vi "FRC Color Processing RetroTape Example.vi"() -> ()   [LabVIEW 2019]
uses:
  <vilib>/Rock Robotics/WPI/Camera/WPI_CameraSettings Read MJPG.ctl
  <vilib>/Rock Robotics/WPI/Camera/WPI_CameraImageSize.ctl
  Vision Support Code/Camera Types.ctl
  <vilib>/Rock Robotics/WPI/Camera/WPI_CameraExposure Values.ctl
  <vilib>/Rock Robotics/WPI/Camera/WPI_CameraWhite Balance Values.ctl
  <vilib>/vision/NI_Vision_Development_Module.lvlib
panel:
  out "Disqualified":i32=13
  out "Results":T1(array[cluster])=[{"diameter points"={"first point"={"x"=213.0, "y"=163.0}, "projected point"={"x"=293.0, "y"=194.0}}, "Normalized Center"={"x"=0.58125, "y"=0.48750000000000004}, "Overall Score"=61.175669724085026, "Area Score"=96.13589211618256, "Moment Score"=62.73202614698161, "Aspect Score"=24.659090909090907, "Distance (ft)"=4.347709612348454, "Upper Goal"=FALSE}, {"diameter points"={"first point"={"x"=243.0, "y"=142.0}, "projected point"={"x"=266.0, "y"=171.0}}, "Normalized Center"={"x"=0.5906250000000002, "y"=0.3041666666666667}, "Overall Score"=74.56623386292142, "Area Score"=82.18546637744035, "Moment Score"=61.2760810611263, "Aspect Score"=80.23715415019763, "Distance (ft)"=15.122468216864188, "Upper Goal"=FALSE}] {"Normalized Center"."x" format="%#_2g"; "Normalized Center"."y" format="%#_2g"; "Overall Score" format="%#_2g"; "Distance (ft)" format="%#_3g"; "Area Score" format="%#_2g"; "Moment Score" format="%#_2g"; "Aspect Score" format="%#_2g"}
  in  "Size Limit %":dbl=0.04 min=0.0 max=100.0 step=0.01 format="%#_13g"
  out "Instructions:":string="Instructions:\nUse Source to load image files from a directory, or use a USB or IP camera connected to your laptop. Use Camera Settings 1 and 2 to achieve a dark image with bright and colorful stripes.\nLED Color can encoded as HSL or related color modes. Calibrate to the same color as the strips being reflected to the camera.\nClick and draw a line in Original Image to auto-calibrate the LED Color. You may want to widen and tweak Sat and Val by hand.\nThe Annotate button affects drawing a rectangle around the stripes and labeling it with a distance in ft. Distance relies on knowing the Camera Type and lens calibration (it looks up the lens view angle).\n\nAdjust Score Cutoff to make the code more or less picky. If the color is not very unique, you may need to increase the number of particles considered. The diagram uses a Size Limit to ignore colored things that are too small. You may need to adjust it if you are targetting from far away.\n\nResults give you the distance to the target, the center and box in a normalized (-1 to 1) and pixel coordinates.\n\nBe sure to read about setting camera exposure and brightness to help simplify your image and acquire color saturated images.\n\nThere are lots of comments on the diagram to explain the code."
  in  "Color Mode":u16(ring)=2 items=["RGB", "HSL", "HSV", "HSI"]
  in  "Particle Count":i32=5
  in  "Score Threshold %":dbl=75.0
  in  "Std Devs for Calibration":cluster{"H":dbl, "S":dbl, "V":dbl}={"H"=4.0, "S"=8.0, "V"=8.0}
  in  "Camera Type (for distance)":T2=enum."MS HD3000 square"
  in  "image files":string[](array[string])=["BlueGoal-060in-Center.jpg", "BlueGoal-084in-Center.jpg", "BlueGoal-108in-Center.jpg", "BlueGoal-132in-Center.jpg", "BlueGoal-156in-Center.jpg", "BlueGoal-156in-Left.jpg", "BlueGoal-180in-Center.jpg", "BlueGoal-224in-Center.jpg", "BlueGoal-228in-ProtectedZone.jpg", "BlueGoal-330in-ProtectedZone.jpg", "BlueGoal-Far-ProtectedZone.jpg", "RedLoading-016in-Down.jpg", "RedLoading-030in-Down.jpg", "RedLoading-048in-Down.jpg", "RedLoading-048in.jpg", "RedLoading-060in.jpg", "RedLoading-084in.jpg", "RedLoading-108in.jpg"]
  in  "Source":enum32{"Files", "Camera"}(tab)=enum."Camera"
  in  "Images":i32(listbox)
  in  "Folder Location":path=path "C:/Users/5052r/Downloads/2020 Vision Example/Dark Images"
  in  "Camera Settings 1":T3={"fps"=20, "compression"=30, "Image Size"=enum."320x240", "Config Shown"=FALSE}
  in  "Camera Address":string="USB 0"
  in  "Camera Settings 2":T7={"Exposure"=enum."Auto", "Exposure (%)"=50.0, "Brightness"=50, "White Balance"=enum."Auto", "Color Temp (K)"=0.0} {"Brightness" min=0 max=100}
  in  "Annotate":bool=TRUE
  out "Qualified":i32=5
  in  "LED Color Range":T8={"Hue"={14.360681298918061, 47.91090746924753}, "Sat"={75.89285714285714, 255.0}, "Val"={97.14285714285714, 251.32874298095703}} {"Hue" scale=0.0..255.0 scale format="%#_3g"}
  out "Mask":T9(plugin-control)
  out "Original Image":T9(plugin-control)
  # "Limits"
  # "Particle Results"
  # "Good target"
  # "Disqualified"
  # "Distance (ft)"
  # "Scores"
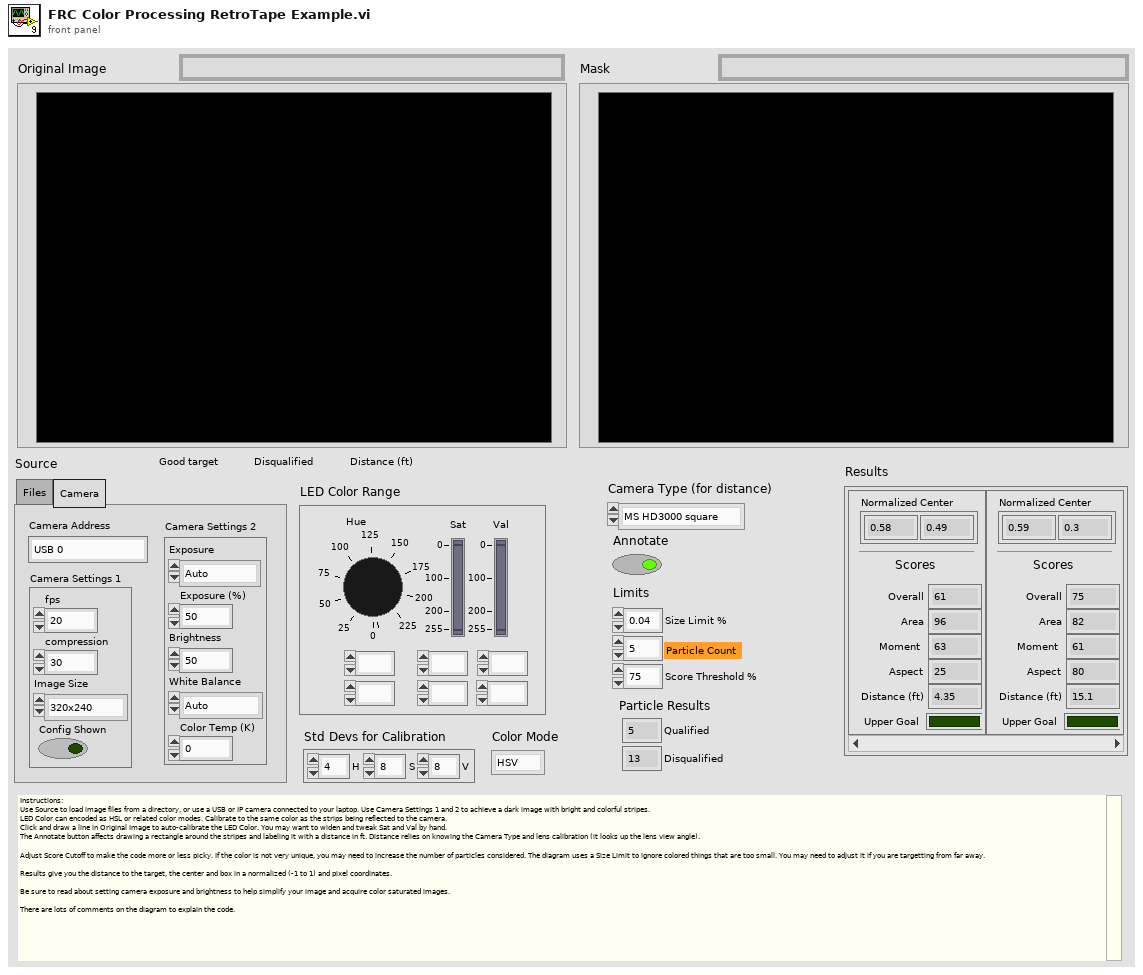
[diagram p1: front panel]
types:
  T1 = cluster{"diameter points":cluster{"first point":cluster{"x":dbl, "y":dbl}, "projected point":cluster{"x":dbl, "y":dbl}}, "Normalized Center":cluster{"x":dbl, "y":dbl}, "Overall Score":dbl, "Area Score":dbl, "Moment Score":dbl, "Aspect Score":dbl, "Distance (ft)":dbl, "Upper Goal":bool}[]
  T2 = typedef "Camera Types.ctl" = enum16{"206", "1011", "1013", "MS HD3000 square", "MS HD3000 640x480"}
  T3 = typedef "WPI_CameraSettings Read MJPG.ctl" = cluster{"fps":i32, "compression":i32, "Image Size":T4, "Config Shown":bool}
  T4 = typedef "WPI_CameraImageSize.ctl" = enum16{"640x480", "320x240", "160x120", "Custom"}
  T5 = typedef "WPI_CameraExposure Values.ctl" = enum16{"Auto", "Flicker-free 50 Hz", "Flicker-free 60 Hz", "Hold current", "Custom"}
  T6 = typedef "WPI_CameraWhite Balance Values.ctl" = enum16{"Auto", "Fixed indoor", "Fixed outdoor 1", "Fixed outdoor 2", "Fixed fluorescent 1", "Fixed fluorescent 2", "Hold current", "Custom"}
  T7 = cluster{"Exposure":T5, "Exposure (%)":dbl, "Brightness":i32, "White Balance":T6, "Color Temp (K)":dbl}
  T8 = cluster{"Hue":cluster{dbl, dbl}, "Sat":cluster{dbl, dbl}, "Val":cluster{dbl, dbl}}
  T9 = typedef "IMAQ Image.ctl" = refnum<image>
  T10 = typedef "Particle Parameters" = i32
  T11 = typedef "Image Type" = u32
  T12 = enum32{"AutoM", "Close", "Dilate", "Erode", "Gradient", "Gradient out", "Gradient in", "Hit miss", "Open", "PClose", "POpen", "Thick", "Thin"}
  T13 = cluster{cluster{dbl, dbl}, cluster{dbl, dbl}, cluster{dbl, dbl}}
  T14 = cluster{"remainder":i32, "size":bool, "count":bool}
  T15 = typedef "Target Fields.ctl" = cluster{"diameter points":cluster{"first point":cluster{"x":dbl, "y":dbl}, "projected point":cluster{"x":dbl, "y":dbl}}, "normalized center":cluster{"x":dbl, "y":dbl}, "Overall Score":dbl, "Area Score":dbl, "Moment Score":dbl, "Aspect Score":dbl, "Distance (ft)":dbl, "Upper Goal":bool}
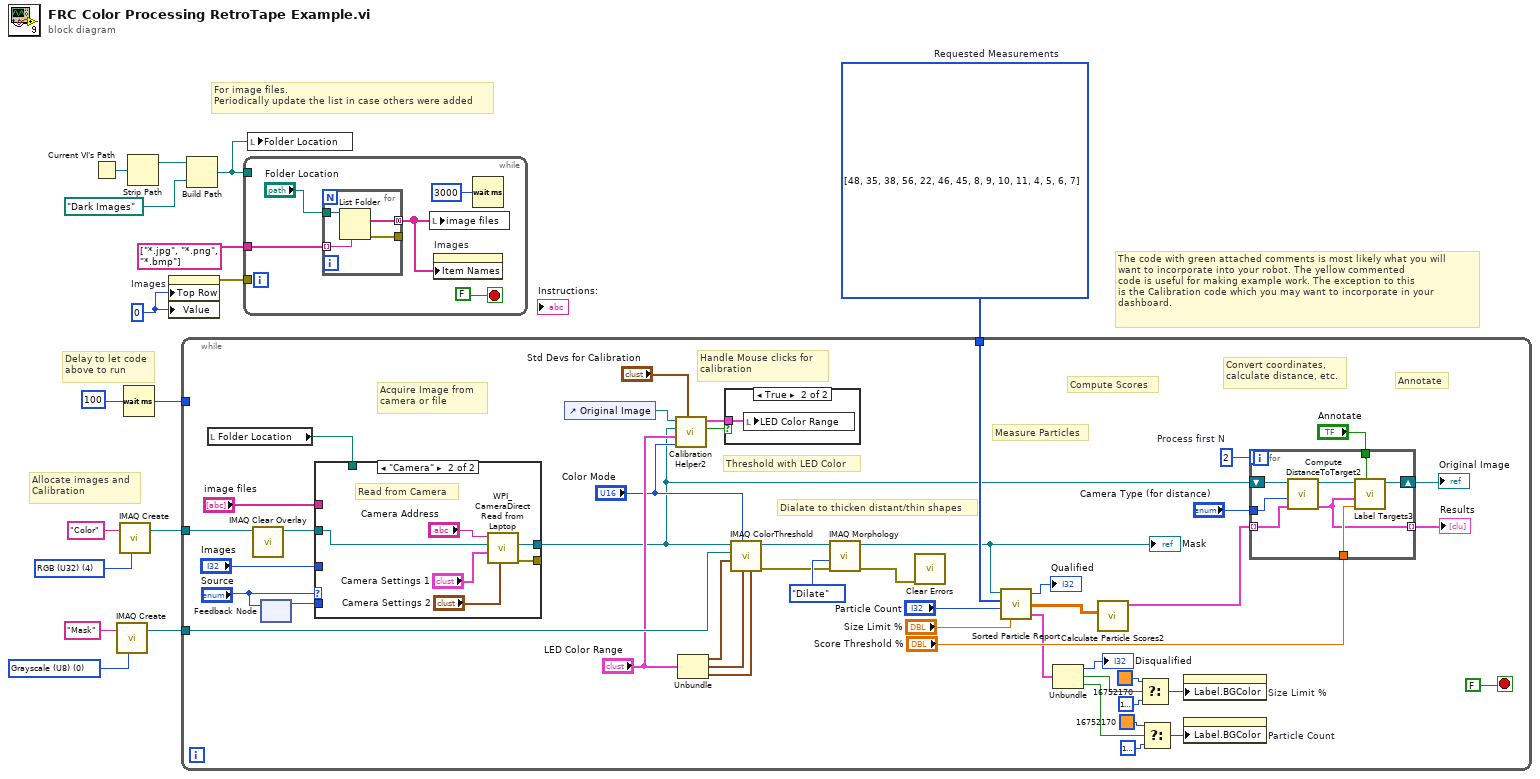
[diagram p0: block diagram]
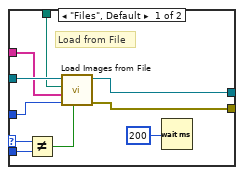
[diagram p3: hidden frame]
diagram:
  w6 = u32 0 ("milliseconds to wait")
  w11 = T10[] [48, 35, 38, 56, 22, 46, 45, 8, 9, 10, 11, 4, 5, 6, 7] items=["Center of Mass X", "Center of Mass Y", "First Pixel X", "First Pixel Y", "Bounding Rect Left", "Bounding Rect Top", "Bounding Rect Right", "Bounding Rect Bottom", "Max Feret Diameter Start X", "Max Feret Diameter Start Y", "Max Feret Diameter End X", "Max Feret Diameter End Y", "Max Horiz. Segment Length Left", "Max Horiz. Segment Length Right", "Max Horiz. Segment Length Row", "-", "Bounding Rect Width", "Bounding Rect Height", "Bounding Rect Diagonal", "Perimeter", "Convex Hull Perimeter", "Holes' Perimeter", "Max Feret Diameter", "Equivalent Ellipse Major Axis", "Equivalent Ellipse Minor Axis", "Equivalent Ellipse Minor Axis (Feret)", "Equivalent Rect Long Side", "Equivalent Rect Short Side", "Equivalent Rect Diagonal", "Equivalent Rect Short Side (Feret)", "Average Horiz. Segment Length", "Average Vert. Segment Length", "Hydraulic Radius", "Waddel Disk Diameter", "-", "Area", "Holes' Area", "Particle & Holes' Area", "Convex Hull Area", "Image Area", "-", "Number of Holes", "Number of Horiz. Segments", "Number of Vert. Segments", "-", "Orientation", "Max Feret Diameter Orientation", "-", "% Area/Image Area", "% Area/(Particle & Holes' Area)", "Ratio of Equivalent Ellipse Axes", "Ratio of Equivalent Rect Sides", "-", "Elongation Factor", "Compactness Factor", "Heywood Circularity Factor", "Type Factor", "-", "Sum X", "Sum Y", "Sum XX", "Sum XY", "Sum YY", "Sum XXX", "Sum XXY", "Sum XYY", "Sum YYY", "-", "Moment of Inertia XX", "Moment of Inertia XY", "Moment of Inertia YY", "Moment of Inertia XXX", "Moment of Inertia XXY", "Moment of Inertia XYY", "Moment of Inertia YYY", "Norm. Moment of Inertia XX", "Norm. Moment of Inertia XY", "Norm. Moment of Inertia YY", "Norm. Moment of Inertia XXX", "Norm. Moment of Inertia XXY", "Norm. Moment of Inertia XYY", "Norm. Moment of Inertia YYY", "Hu Moment 1", "Hu Moment 2", "Hu Moment 3", "Hu Moment 4", "Hu Moment 5", "Hu Moment 6", "Hu Moment 7"]  # Requested Measurements
  w14 = T11 0 items=["Grayscale (U8)", "Grayscale (I16)", "Grayscale (SGL)", "Complex (CSG)", "RGB (U32)", "HSL (U32)", "RGB (U64)", "Grayscale (U16)"] ("Image Type")
  w15 = T11 4 items=["Grayscale (U8)", "Grayscale (I16)", "Grayscale (SGL)", "Complex (CSG)", "RGB (U32)", "HSL (U32)", "RGB (U64)", "Grayscale (U16)"] ("Image Type")
  # "Delay to let code\nabove to run"
  # "The code with green attached comments is most likely what you will\nwant to incorporate into your robot. The yellow commented\ncode is useful for making example work. The exception to this\nis the Calibration code which you may want to incorporate in your\ndashboard."
  # "For image files.\nPeriodically update the list in case others were added"
  # "Allocate images and\nCalibration"
  n1 = Current VI's Path() -> (path=w10:path)
  n2 = call "IMAQ Create"("Image Name"="Mask", "Image Type"=w14) -> ("New Image"=w12:T9)  [unwired: 2 in, 2 out]
  n3 = call "IMAQ Create"("Image Name"="Color", "Image Type"=w15) -> ("New Image"=w4:T9)  [unwired: 2 in, 2 out]
  n4 = Wait (ms)(milliseconds to wait=u32 100) -> (millisecond timer value=w2:u32)
  n5 = Strip Path(path=w10) -> (stripped path=w8:path)  [unwired: 1 out]
  n6 = property on="Images" class="LstBox (strict)"("Top Row"=w6, "Value"=w6) -> (error out=w7:errorcluster)  [unwired: 2 in, 1 out]
  n7 = while {
    tunnel: w4 -> [w37]
    tunnel: w12 -> [w60]
    tunnel: w11 -> [w56]
    tunnel: w2 -> [_]
    stop <- FALSE stop-if-true
    w39 = 2  # Process first N
    # "Dialate to thicken distant/thin shapes"
    # "Handle Mouse clicks for\ncalibration"
    # "Measure Particles"
    # "Convert coordinates,\ncalculate distance, etc."
    # "Annotate"
    # "Compute Scores"
    # "Threshold with LED Color"
    # "Acquire Image from\ncamera or file"
    n8 = local read "Folder Location"() -> (w47:path)
    n9 = call "IMAQ Clear Overlay"("Image"=w37) -> ("Image Out"=w36:T9)  [unwired: 2 in, 8 out]
    n10 = feedback #1() -> (w45:enum32{"Files", "Camera"})  [unwired: 1 in]
    n11 = feedback-in #1("Source") -> ()
    n12 = case shown="\"Camera\"" "Source" {
      selector: "Source" -> [w74 _]
      tunnel: [w80 w87] -> _
      tunnel: [w81 w86] -> w38
      tunnel: w36 -> [w79 w85]
      tunnel: "image files" -> [w76 _]
      tunnel: "Images" -> [w78 _]
      tunnel: w47 -> [w77 _]
      tunnel: w45 -> [w73 _]
      frame "Files", Default {
        # "Load from File"
        n13 = Not Equal?(x=w74, y=w73) -> (x != y?=w72:bool)
        n14 = call "Load Images from File.vi"("Force Load"=w72, "Images"=w78, "image files"=w76, "Folder Location"=w77, "Refnum in"=w79) -> ("error out"=w80:errorcluster, "Refnum out"=w81:T9)  [unwired: 4 in, 1 out]
        n15 = Wait (ms)(milliseconds to wait=u32 200 ("delay (ms)")) -> ()  [unwired: 1 out]
      }
      frame "Camera" {
        # "Read from Camera"
        n16 = call <vilib>:"WPI_CameraDirect Read from Laptop.vi"("Camera Settings 2"="Camera Settings 2", "Camera Settings"="Camera Settings 1", "Image"=w85, "address"="Camera Address") -> ("error out"=w87:errorcluster, "Image Out"=w86:T9)  [unwired: 6 in]
      }
    }
    n17 = control-ref of="Original Image"() -> (w52:refnum<vi>)
    n18 = call "Calibration Helper2.vi"("Std Devs"="Std Devs for Calibration", "Color Mode"="Color Mode", "Color Components"="LED Color Range", "Image"=w38, "Image Ctl Refnum"=w52) -> ("Changed"=w51:bool, "output color"=w50:T13)  [unwired: 5 in]
    n19 = Unbundle("LED Color Range") -> ("Hue"=w59:cluster{dbl, dbl}, "Sat"=w58:cluster{dbl, dbl}, "Val"=w57:cluster{dbl, dbl})
    n20 = case shown="True" w51 {
      tunnel: w50 -> [_ w71]
      frame False {
      }
      frame True {
        n21 = local write "LED Color Range"(w71) -> ()
      }
    }
    n22 = call "IMAQ ColorThreshold"("Blue or Luma or Val or Inten Range"=w57, "Green or Sat Range"=w58, "Color Mode"="Color Mode", "Red or Hue Range"=w59, "Image Dst"=w60, "Image Src"=w38) -> ("error out"=w33:errorcluster, "Image Dst Out"=w35:T9)  [unwired: 4 in]
    n23 = call "IMAQ Morphology"("error in (no error)"=w33, "Operation"=T12."Dilate", "Image Src"=w35) -> ("error out"=w32:errorcluster, "Image Dst Out"=w29:T9)  [unwired: 7 in]
    "Mask" <- w29
    n24 = call <vilib>:"Clear Errors.vi"("error in (no error)"=w32) -> ()  [unwired: 5 in, 2 out]
    n25 = call "Sorted Particle Report.vi"("Min Area Size %"="Size Limit %", "Particle Count Limit"="Particle Count", "Pixel Measurements"=w56, "Image in"=w29) -> ("limits"=w26:T14, "Sorted Data"=w31:dbl[][], "Particles"=→"Qualified":i32)
    n26 = Unbundle(w26) -> ("remainder"=→"Disqualified":i32, "size"=w20:bool, "count"=w19:bool)
    n27 = call "Calculate Particle Scores2.vi"("Sorted Data"=w31) -> ("Scores"=w30:T15[])  [unwired: 10 in]
    n28 = Select(t=u32 16752170 ("Color"), s=w20, f=u32 16777216 ("Color")) -> (s? t:f=w18:u32)
    n29 = Select(t=u32 16752170 ("Color"), s=w19, f=u32 16777216 ("Color")) -> (s? t:f=w17:u32)
    n30 = property on="Size Limit %" class="DigNum (strict)"("Label.BGColor"=w18) -> ()  [unwired: 2 in, 2 out]
    n31 = property on="Particle Count" class="DigNum (strict)"("Label.BGColor"=w17) -> ()  [unwired: 2 in, 2 out]
    n32 = for {
      N: w39 -> [_]
      tunnel: w30 -> [w68] mode=indexing
      tunnel: "Camera Type (for distance)" -> [w70]
      tunnel: "Annotate" -> [w65]
      shift-right: [w69] -> w40
      shift-left: w38 -> [w67]
      tunnel: "Score Threshold %" -> [w64]
      tunnel: [w63] -> w27 mode=indexing
      n33 = call "Compute DistanceToTarget2.vi"("results"=w68, "Camera Type"=w70, "Image Src"=w67) -> ("results out"=w63:T15, "Image Dst Out"=w66:T9)  [unwired: 7 in]
      n34 = call "Label Targets3.vi"("Annotate"=w65, "Score Threshold"=w64, "results"=w63, "Image in"=w66) -> ("Image out"=w69:T9)  [unwired: 7 in]
    }
    "Original Image" <- w40
    "Results" <- w27
  }
  n35 = Build Path(base path=w8, name or relative path=path "Dark Images" ("Folder Location")) -> (appended path=w3:path)
  n36 = while {
    tunnel: w3 -> [_]
    tunnel: w7 -> [_]
    tunnel: string[] ["*.jpg", "*.png", "*.bmp"] -> [w88]
    stop <- FALSE stop-if-true
    n37 = for {
      tunnel: [w96] -> w90 mode=concatenating
      tunnel: "Folder Location" -> [w95]
      tunnel: [w94] -> _
      tunnel: w88 -> [w93] mode=indexing
      n38 = List Folder(path=w95, pattern=w93) -> (filenames=w96:string[], error out=w94:errorcluster)  [unwired: 2 in, 2 out]
    }
    n39 = local write "image files"(w90) -> ()
    n40 = property on="Images" class="LstBox (strict)"("Item Names"=w90) -> ()  [unwired: 2 in, 2 out]
    n41 = Wait (ms)(milliseconds to wait=u32 3000) -> ()  [unwired: 1 out]
  }
  n42 = local write "Folder Location"(w3) -> ()
